vi "Convert Temp 1D to 2D.vi"(6 "Width":i32, 7 "Height":i32, 8 "error in (no error)":errorcluster, 10 "Temperatures (C)":dbl[](array[numeric]), 11 "Optris PI in":refnum<class "Optris PI.lvclass">) -> (0 "error out":errorcluster, 2 "Area Temps":dbl[][](array[numeric]), 3 "Optris PI out":refnum<class "Optris PI.lvclass">)   [LabVIEW 2018, in "Optris PI.lvlib" / "Optris PI.lvclass"]
uses:
  Optris PI.lvclass
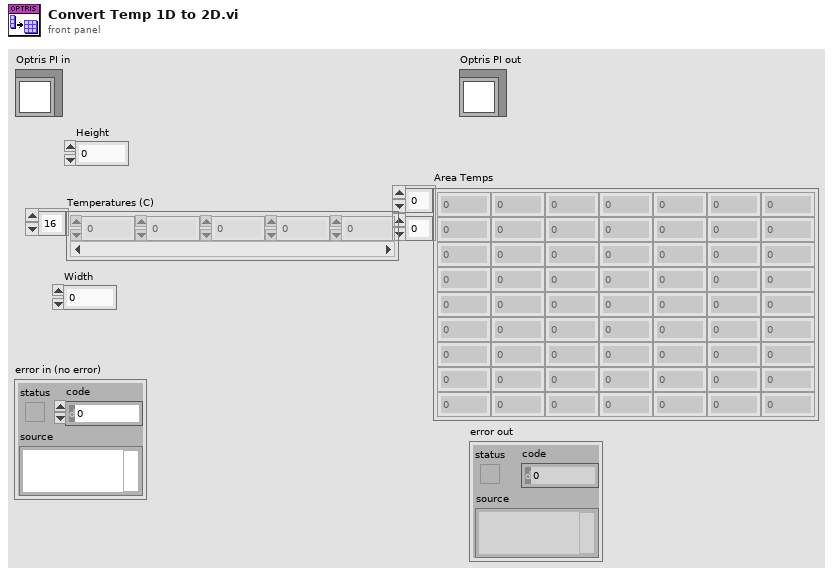
[diagram p1: front panel]
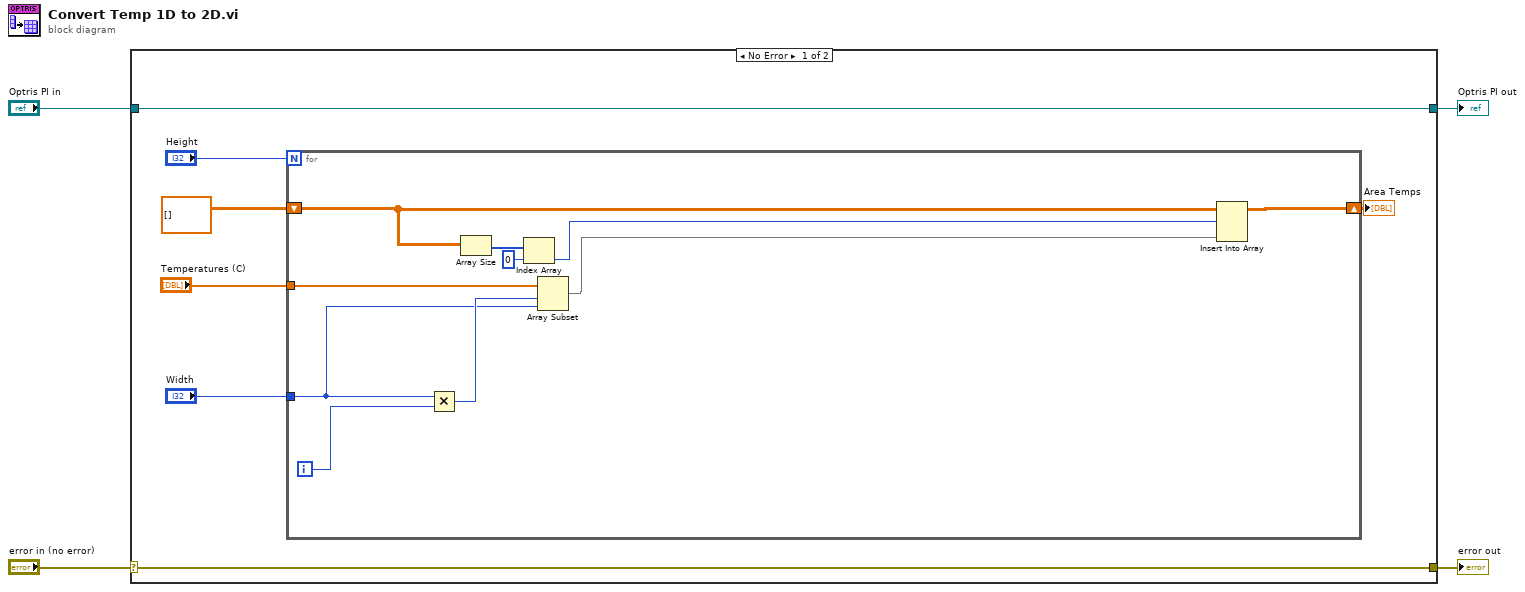
[diagram p0: block diagram]
diagram:
  n1 = case shown="No Error" "error in (no error)" {
    selector: "error in (no error)" -> [w10 w23]
    tunnel: [w10 w23] -> w3
    tunnel: [w11 w22] -> w1
    tunnel: "Optris PI in" -> [w11 w22]
    frame No Error {
      n2 = for {
        N: "Height" -> [_]
        shift-right: [w12] -> w5
        shift-left: dbl[][] [] ("Area Temps") -> [w16]
        tunnel: "Temperatures (C)" -> [w20]
        tunnel: "Width" -> [w13]
        i -> [w21]
        n3 = Multiply(x=w13, y=w21) -> (x*y=w19:i32)
        n4 = Array Size(array=w16) -> (size(s)=w18:i32[])
        n5 = Index Array(array=w18, index=0) -> (element=w15:i32)
        n6 = Array Subset(array=w20, index=w19, length=w13) -> (w14:dbl[])
        n7 = Insert Into Array(array=w16, index (row)=w15, new element=w14) -> (w12:dbl[][])  [unwired: 1 in]
      }
      "Area Temps" <- w5
    }
    frame Error {
    }
  }
  "error out" <- w3
  "Optris PI out" <- w1
